vi "Test 2.vi"(2 "Dynamic Data Type":dynamicdata(graph)) -> (4 "Array of Waveform":waveform(dbl)[](array[waveform]))   [LabVIEW 2021]
doc: "Converts the dynamic data type to numeric, Boolean, waveform, and array data types for use with other VIs and functions."
uses:
  Illuminace (SubVI).vi
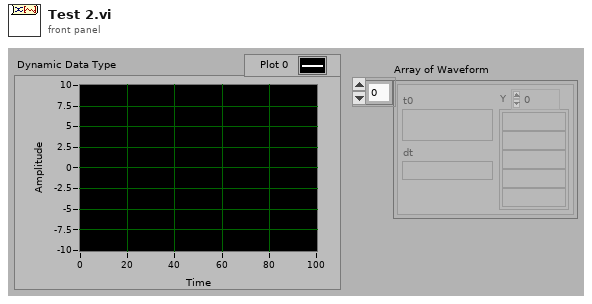
[diagram p1: front panel]
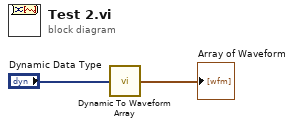
[diagram p0: block diagram]
diagram:
  n1 = call <vilib>:"Dynamic To Waveform Array.vi"("Input"="Dynamic Data Type") -> ("Output"=→"Array of Waveform":waveform(dbl)[])  [unwired: 4 in]
